vi "Image Cap Get Serial Number.vi"(8 "error in (no error)":errorcluster, 10 "lpszSerialNum":string, 11 "nSensorIP":u32) -> (0 "error out":errorcluster, 2 "lpszSerialNum out":string, 3 "function return":i32)   [LabVIEW 2017, in "BonTechDetector.lvlib"]
doc: "DLLFunction int __stdcall ImageCapGetSerialNumber(unsigned int nSensorIP, LPTSTR lpszSerialNum);"
uses:
  BonTechDetector.lvlib
  lib/ImageCaptureDLL.dll
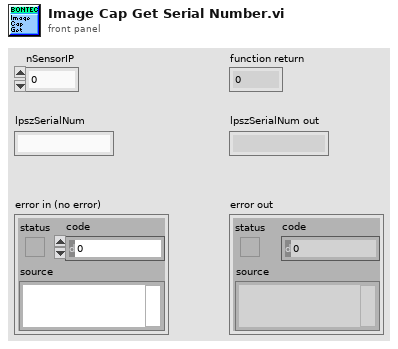
[diagram p1: front panel]
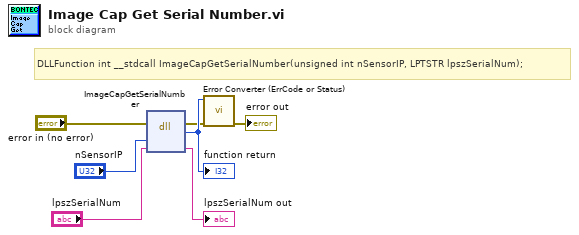
[diagram p0: block diagram]
diagram:
  # "DLLFunction int __stdcall ImageCapGetSerialNumber(unsigned int nSensorIP, LPTSTR lpszSerialNum);"
  n1 = dll-call lib="F:/BonTechFlatPanelLVDriver/lib/ImageCaptureDLL.*" fn="ImageCapGetSerialNumber"(error in="error in (no error)", "nSensorIP"="nSensorIP", "lpszSerialNum"="lpszSerialNum") -> (error out=w2:errorcluster, w7:i32, "lpszSerialNum"=→"lpszSerialNum out":string)  [unwired: 3 in, 1 out]
  "function return" <- w7
  n2 = call "Error Converter (ErrCode or Status).vi"("error in (no error)"=w2, "error code"=w7) -> ("error out"=→"error out":errorcluster)  [unwired: 9 in]
